vi "Plot Curves.vi"(6 "Ctl Refnum":refnum<vi>, 7 "RPM info":cluster{"smallest":dbl, "resolution":dbl} {"resolution" format="%.2f"; "smallest" format="%.2f"}, 8 "ColorMapStyle":i32(ring) items=["cwNone", "cwShaded", "cwColorSpectrum", "cwGrayScale"], 9 "Order array":dbl[](array[numeric]) format="%.2f", 10 "orders":u8[][](array[numeric]), 11 "orders":refnum<k7>) -> ()   [LabVIEW 2017]
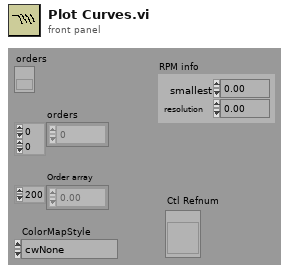
[diagram p1: front panel]
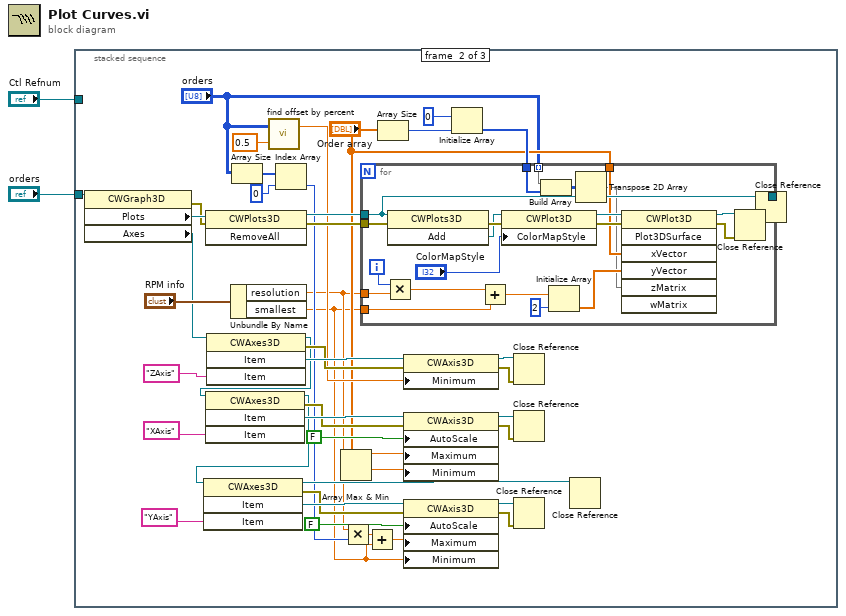
[diagram p0: block diagram]
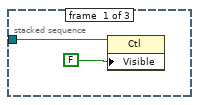
[diagram p2: hidden frame]
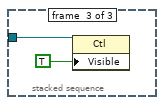
[diagram p3: hidden frame]
diagram:
  n1 = stacked-sequence {
    tunnel: "orders" -> [_ w42 _]
    tunnel: "Ctl Refnum" -> [w3 _ w70]
    frame #0 {
      n2 = property class="Ctl"(reference=w3, "Visible"=FALSE ("Defer Panel Updates")) -> ()  [unwired: 1 in, 2 out]
    }
    frame #1 {
      n3 = property class="CWGraph3D"(reference=w42) -> (error out=w45:errorcluster, "Plots"=w46:refnum<k7>, "Axes"=w26:refnum<k7>)  [unwired: 1 in, 1 out]
      n4 = invoke class="CWPlots3D" method="RemoveAll"(reference=w46, error in=w45) -> (reference out=w47:refnum<k7>, error out=w44:errorcluster)  [unwired: 1 in, 1 out]
      n5 = invoke class="CWAxes3D" method="Item"(reference=w26, "Item"="ZAxis") -> (reference out=w27:refnum<k7>, error out=w36:errorcluster, "Item"=w39:refnum<k7>)  [unwired: 2 in, 1 out]
      n6 = invoke class="CWAxes3D" method="Item"(reference=w27, "Item"="XAxis") -> (reference out=w15:refnum<k7>, error out=w30:errorcluster, "Item"=w32:refnum<k7>)  [unwired: 2 in, 1 out]
      n7 = invoke class="CWAxes3D" method="Item"(reference=w15, "Item"="YAxis") -> (reference out=w14:refnum<k7>, error out=w13:errorcluster, "Item"=w16:refnum<k7>)  [unwired: 2 in, 1 out]
      n8 = Unbundle By Name("RPM info") -> ("resolution"=w9:dbl, "smallest"=w5:dbl)
      n9 = Array Size(array="orders") -> (size(s)=w11:i32[])
      n10 = call <vilib>:"find offset by percent.vi"("low %"=0.5, "orders"="orders") -> ("offset"=w35:dbl)  [unwired: 1 in]
      n11 = Index Array(array=w11, index=0) -> (element=w10:i32)
      n12 = Array Max & Min(array="Order array") -> (max value=w24:dbl, min value=w23:dbl)  [unwired: 2 out]
      n13 = Multiply(x=w9, y=w10) -> (x*y=w6:dbl)
      n14 = Add(x=w6, y=w5) -> (x+y=w7:dbl)
      n15 = Array Size(array="Order array") -> (size(s)=w33:i32)
      n16 = property class="CWAxis3D"(reference=w39, error in=w36, "Minimum"=w35) -> (reference out=w37:refnum<k7>, error out=w38:errorcluster)
      n17 = property class="CWAxis3D"(reference=w32, error in=w30, "AutoScale"=FALSE, "Maximum"=w24, "Minimum"=w23) -> (reference out=w29:refnum<k7>, error out=w28:errorcluster)
      n18 = property class="CWAxis3D"(reference=w16, error in=w13, "AutoScale"=FALSE, "Maximum"=w7, "Minimum"=w5) -> (reference out=w18:refnum<k7>, error out=w19:errorcluster)
      n19 = Initialize Array(u8 0 ("Element Data"), w33) -> (w48:u8[])
      n20 = for {
        tunnel: "orders" -> [w53] mode=indexing
        tunnel: w48 -> [w52]
        tunnel: w47 -> [w60]
        tunnel: "Order array" -> [w51]
        tunnel: w44 -> [w61]
        tunnel: [w60] -> w43
        tunnel: w9 -> [w56]
        tunnel: w5 -> [w55]
        i -> [w64]
        n21 = Multiply(x=w64, y=w56) -> (x*y=w57:dbl)
        n22 = invoke class="CWPlots3D" method="Add"(reference=w60, error in=w61) -> (error out=w66:errorcluster, "Add"=w63:refnum<k7>)  [unwired: 1 in, 1 out]
        n23 = Add(x=w57, y=w55) -> (x+y=w69:dbl)
        n24 = property class="CWPlot3D"(reference=w63, error in=w66, "ColorMapStyle"="ColorMapStyle") -> (reference out=w62:refnum<k7>, error out=w65:errorcluster)
        n25 = Build Array(w53, w52) -> (w54:u8[][])
        n26 = Initialize Array(w69, 2 ("Dimension Size")) -> (w50:dbl[])
        n27 = Transpose 2D Array(2D array=w54) -> (transposed array=w49:u8[][])
        n28 = invoke class="CWPlot3D" method="Plot3DSurface"(reference=w62, error in=w65, "xVector"=w51, "yVector"=w50, "zMatrix"=w49) -> (reference out=w59:refnum<k7>, error out=w58:errorcluster)  [unwired: 2 in, 5 out]
        n29 = Close Reference(reference=w59, error in (no error)=w58) -> ()  [unwired: 1 out]
      }
      n30 = Close Reference(reference=w37, error in (no error)=w38) -> ()  [unwired: 1 out]
      n31 = Close Reference(reference=w29, error in (no error)=w28) -> ()  [unwired: 1 out]
      n32 = Close Reference(reference=w18, error in (no error)=w19) -> ()  [unwired: 1 out]
      n33 = Close Reference(reference=w14) -> ()  [unwired: 1 in, 1 out]
      n34 = Close Reference(reference=w43) -> ()  [unwired: 1 in, 1 out]
    }
    frame #2 {
      n35 = property class="Ctl"(reference=w70, "Visible"=TRUE ("Defer Panel Updates")) -> ()  [unwired: 1 in, 2 out]
    }
  }
